vi "Perform Work.vi"(6 "Last request":bool, 8 "error in (no error)":errorcluster, 9 "Initialize":bool, 10 "Reply to":refnum<class "Result Reply Msg.lvclass">, 11 "Timer in":refnum<class "Timer.lvclass">) -> (0 "error out":errorcluster, 3 "Timer out":refnum<class "Timer.lvclass">)   [LabVIEW 2016, in "Timer.lvclass"]
uses:
  Timer.lvclass
  C:/github/LabActor/Worker/Worker.lvclass
  C:/Program Files (x86)/National Instruments/LabVIEW 2016/vi.lib/ActorFramework/Actor/Actor.lvclass
  Template Module Messages/Result Reply Msg/Result Reply Msg.lvclass
  Timer.lvclass/Timer.ctl
  Worker/Worker.lvclass/Worker.ctl
  <vilib>/ActorFramework/Actor/Actor.lvclass/Actor.ctl
  <vilib>/ActorFramework/Message Enqueuer/Message Enqueuer.lvclass/Message Enqueuer.ctl
  Read Start time.vi
  Worker/Read Cycle period.vi
  Write Latest time.vi
  <vilib>/ActorFramework/Message Enqueuer/Init from Existing Queue.vi
  Timer Messages/Time-Delayed Response Msg/Time-Delayed Response Msg.lvclass
  C:/Program Files (x86)/National Instruments/LabVIEW 2016/vi.lib/ActorFramework/Message/Message.lvclass
  <vilib>/ActorFramework/Time-Delayed Send Message/Time-Delayed Send Message.vi
  Worker/Worker.lvclass
  <vilib>/ActorFramework/Message Enqueuer/Message Enqueuer.lvclass
  <vilib>/ActorFramework/Actor/Actor.lvclass
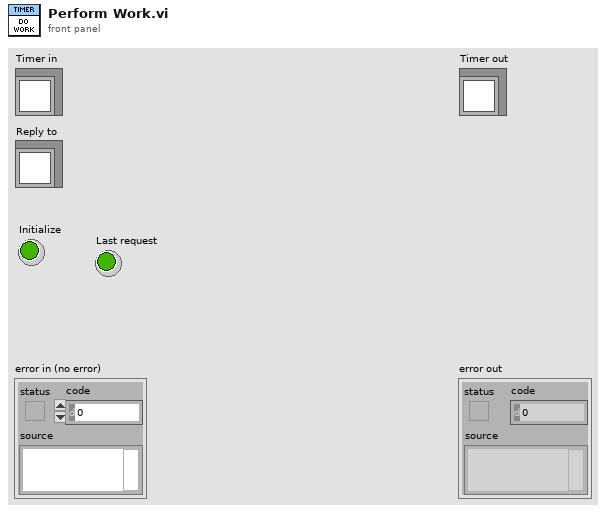
[diagram p1: front panel]
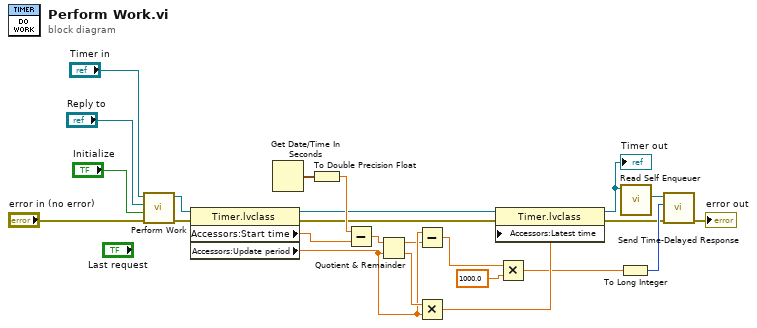
[diagram p0: block diagram]
diagram:
  n1 = call-parent "Perform Work.vi"("error in (no error)"="error in (no error)", "Initialize"="Initialize", "Reply to"="Reply to", "Measure Object in"="Timer in") -> ("error out"=w14:errorcluster, "Measure Object out"=w24:refnum<class "Timer.lvclass">)  [unwired: 6 in]
  n2 = property class="Timer.lvclass"(reference=w24, error in=w14) -> (reference out=w8:refnum<class "Timer.lvclass">, error out=w3:errorcluster, "Accessors:Start time"=w19:dbl, "Accessors:Update period"=w12:dbl)
  n3 = Get Date/Time In Seconds() -> (seconds since 1Jan1904=w18:timestamp)
  n4 = To Double Precision Float(number=w18) -> (double precision float=w17:dbl)
  n5 = Subtract(x=w17, y=w19) -> (x-y=w16:dbl)
  n6 = Quotient & Remainder(x=w16, y=w12) -> (x-y*floor(x/y)=w11:dbl, floor(x/y)=w13:dbl)
  n7 = Subtract(x=w12, y=w11) -> (x-y=w10:dbl)
  n8 = Multiply(x=w13, y=w12) -> (x*y=w15:dbl)
  n9 = property class="Timer.lvclass"(reference=w8, error in=w3, "Accessors:Latest time"=w15) -> (reference out=w1:refnum<class "Timer.lvclass">, error out=w4:errorcluster)
  "Timer out" <- w1
  n10 = Multiply(x=w10, y=1000.0) -> (x*y=w7:dbl)
  n11 = To Long Integer(number=w7) -> (32bit integer=w6:i32)
  n12 = call <vilib>:"Read Self Enqueuer.vi"("Actor"=w1) -> ("Self Enqueuer"=w5:refnum<class "Message Enqueuer.lvclass">)  [unwired: 10 in]
  n13 = call "Send Time-Delayed Response.vi"("error in (no error)"=w4, "Milliseconds To Wait"=w6, "Message Enqueuer"=w5) -> ("error out"=→"error out":errorcluster)  [unwired: 7 in, 1 out]
